vi "Measure_OutPut.vi"(8 "error in (no error)":errorcluster, 10 "Ring":u16(ring) items=["Voltage", "Current", "Power"], 11 "Instrument In":refnum<visa-resource-name>) -> (0 "error out":errorcluster, 2 "Measurement":dbl format="%.4g", 3 "Instrument Out":refnum<visa-resource-name>)   [LabVIEW 2023]
uses:
  <instrlib>/Agilent E363X Series/Agilent E363X Series.lvlib
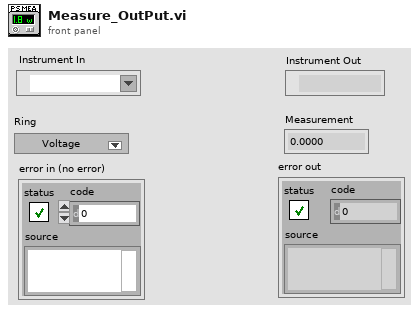
[diagram p1: front panel]
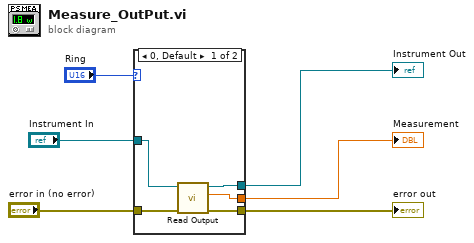
[diagram p0: block diagram]
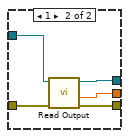
[diagram p2: hidden frame]
diagram:
  n1 = case shown="0, Default" "Ring" {
    tunnel: [w11 w16] -> w6
    tunnel: "error in (no error)" -> [w10 w14]
    tunnel: [w7 w15] -> w1
    tunnel: "Instrument In" -> [w9 w13]
    tunnel: [w8 w12] -> w2
    frame 0, Default {
      n2 = call <instrlib>:"Read Output.vi"("error in (no error)"=w10, "VISA resource name"=w9) -> ("error out"=w11:errorcluster, "Actual Voltage Level (V)"=w7:dbl, "VISA resource name out"=w8:refnum<visa-resource-name>)  [unwired: 6 in, 1 out]
    }
    frame 1 {
      n3 = call <instrlib>:"Read Output.vi"("error in (no error)"=w14, "VISA resource name"=w13) -> ("error out"=w16:errorcluster, "Actual Current Level (A)"=w15:dbl, "VISA resource name out"=w12:refnum<visa-resource-name>)  [unwired: 6 in, 1 out]
    }
  }
  "Instrument Out" <- w2
  "error out" <- w6
  "Measurement" <- w1
